vi "Boost!.vi"(6 "Boost Ctrl":bool, 8 "Normal Factor":dbl, 9 "Boost Factor":dbl, 10 "Axis(y)":dbl, 11 "Axis(x)":dbl) -> (2 "Motor Out(y)":dbl, 3 "Motor Out(x)":dbl)   [LabVIEW 2011]
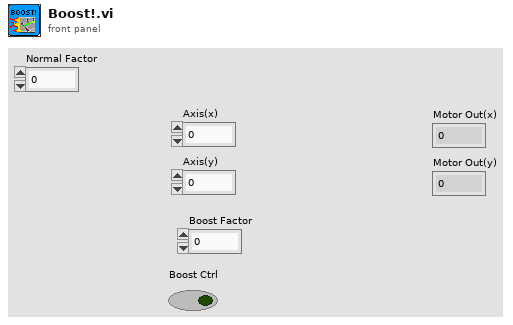
[diagram p1: front panel]
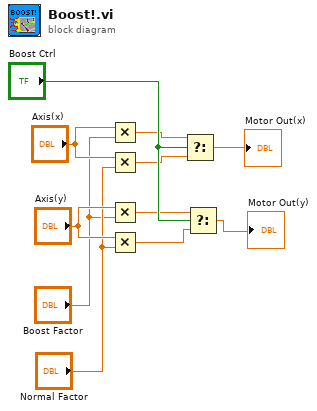
[diagram p0: block diagram]
diagram:
  n1 = Multiply(x="Axis(x)", y="Boost Factor") -> (x*y=w10:dbl)
  n2 = Multiply(x="Axis(x)", y="Normal Factor") -> (x*y=w9:dbl)
  n3 = Multiply(x="Axis(y)", y="Boost Factor") -> (x*y=w3:dbl)
  n4 = Multiply(x="Axis(y)", y="Normal Factor") -> (x*y=w2:dbl)
  n5 = Select(t=w10, s="Boost Ctrl", f=w9) -> (s? t:f=→"Motor Out(x)":dbl)
  n6 = Select(t=w3, s="Boost Ctrl", f=w2) -> (s? t:f=→"Motor Out(y)":dbl)
